vi "DrawCalendar.vi"(8 "error in (no error)":errorcluster, 11 "Calendar in":refnum<class "Calendar.lvclass">) -> (0 "error out":errorcluster, 3 "Calendar out":refnum<class "Calendar.lvclass">)   [LabVIEW 2020, in "Calendar.lvclass"]
uses:
  Calendar.lvclass
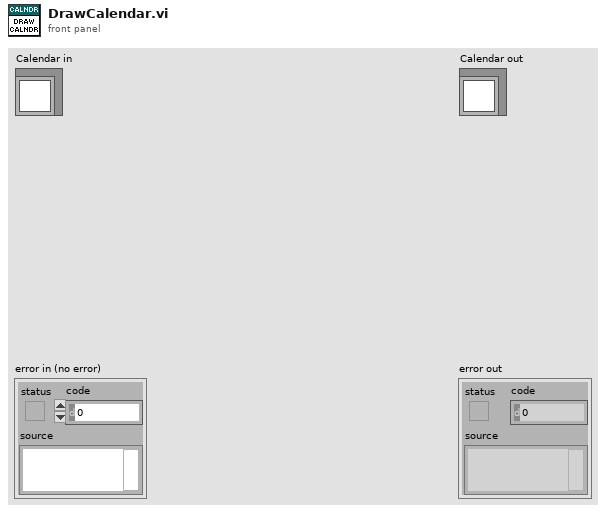
[diagram p1: front panel]
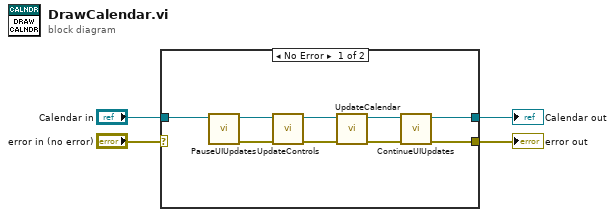
[diagram p0: block diagram]
diagram:
  n1 = case shown="No Error" "error in (no error)" {
    selector: "error in (no error)" -> [_ w15]
    tunnel: [w7 w15] -> w3
    tunnel: [w5 w14] -> w1
    tunnel: "Calendar in" -> [w13 w14]
    frame No Error {
      n2 = call "PauseUIUpdates.vi"("Calendar in"=w13) -> ("error out"=w11:errorcluster, "Calendar out"=w12:refnum<class "Calendar.lvclass">)  [unwired: 9 in]
      n3 = call "UpdateControls.vi"("error in (no error)"=w11, "Calendar in"=w12) -> ("error out"=w9:errorcluster, "Calendar (dup)"=w10:refnum<class "Calendar.lvclass">)  [unwired: 8 in]
      n4 = call "UpdateCalendar.vi"("error in (no error)"=w9, "Calendar in"=w10) -> ("error out"=w8:errorcluster, "Calendar out"=w6:refnum<class "Calendar.lvclass">)  [unwired: 8 in]
      n5 = call "ContinueUIUpdates.vi"("error in (no error)"=w8, "Calendar in"=w6) -> ("error out"=w7:errorcluster, "Calendar out"=w5:refnum<class "Calendar.lvclass">)  [unwired: 8 in]
    }
    frame Error {
    }
  }
  "error out" <- w3
  "Calendar out" <- w1
